vi "Circle Area Perimeter.vi"() -> ()   [LabVIEW 2025]
panel:
  out "Perimeter":dbl
  out "Area":dbl
  in  "r":dbl
  # "ME 235: Design of Microprocessor Based Mechanical Systems"
  # "Lab 1 - Circle Area Perimeter"
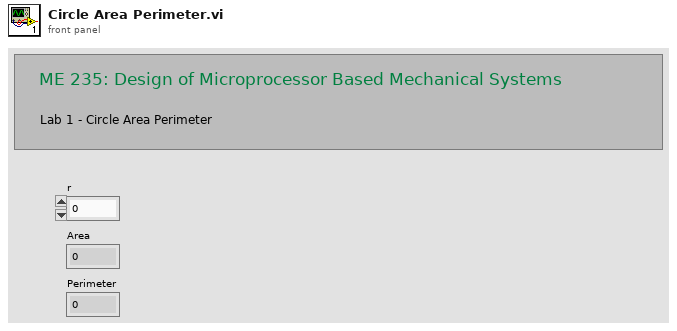
[diagram p1: front panel]
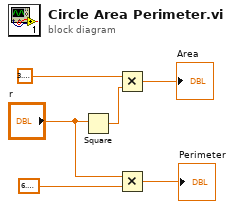
[diagram p0: block diagram]
diagram:
  n1 = Square(x="r") -> (x^2=w1:dbl)
  n2 = Multiply(x=3.141592653589793, y=w1) -> (x*y=→"Area":dbl)
  n3 = Multiply(x="r", y=6.283185307179586) -> (x*y=→"Perimeter":dbl)
